vi "getROI.vi"() -> ()   [LabVIEW 2023]
uses:
  <vilib>/vision/NI_Vision_Development_Module.lvlib
panel:
  out "Inverted":T1(plugin-control)
  out "RemoveBorder":T1(plugin-control)
  out "FillHoles":T1(plugin-control)
  out "Threshold":T1(plugin-control)
  in  "Range":cluster{"Lower value":sgl, "Upper value":sgl}={"Lower value"=128.0, "Upper value"=255.0} {"Upper value" format="%.2f"; "Lower value" format="%.2f"}
  out "Ojo Derecho":T1(plugin-control)
  out "error out 3":errorcluster
  out "error out 2":errorcluster
  out "error out":errorcluster
  out "Ojo Izquierdo":T1(plugin-control)
  out "Image 1":T1(plugin-control)
  in  "stop":bool
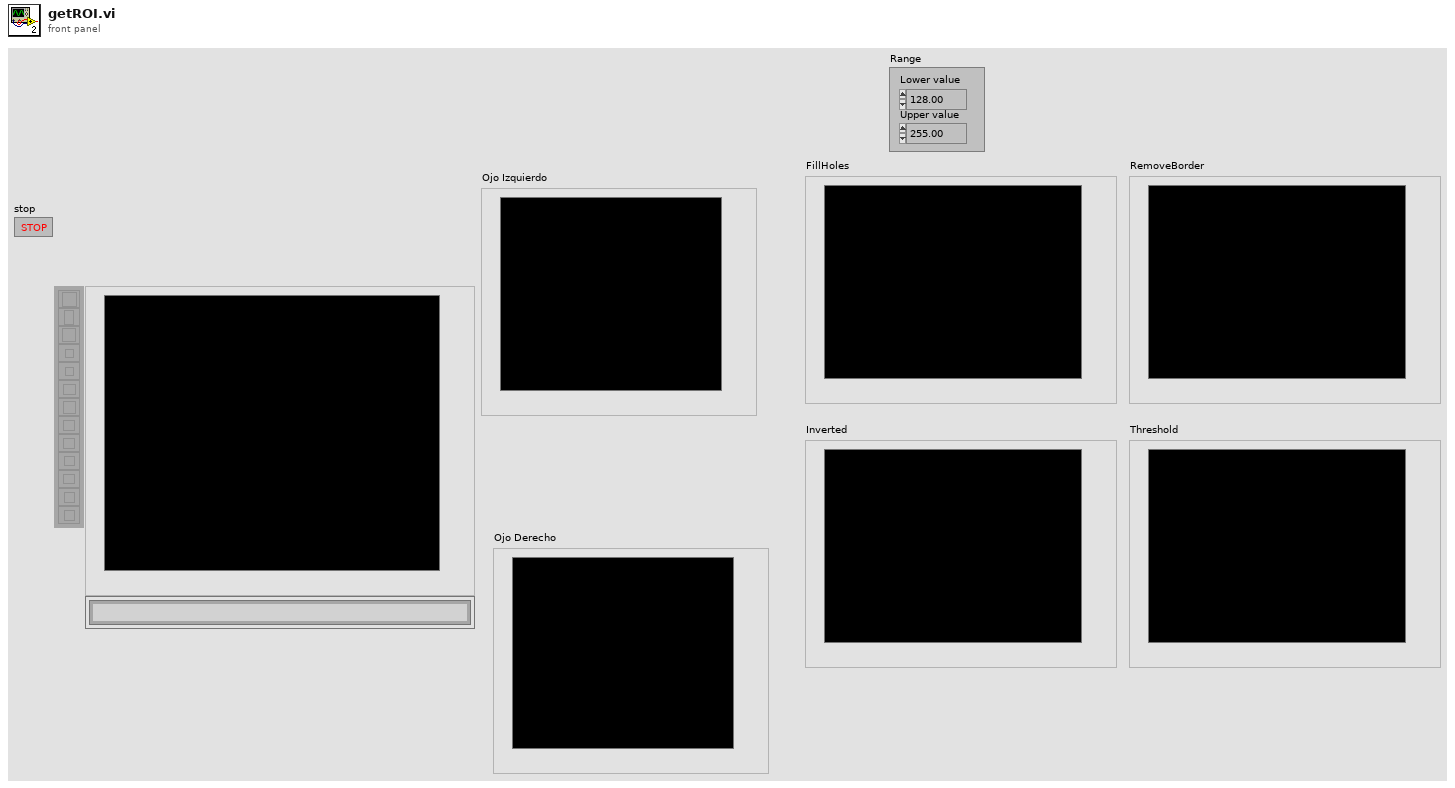
[diagram p1: front panel]
types:
  T1 = typedef "IMAQ Image.ctl" = refnum<image>
  T2 = typedef "Image Type" = u32
  T3 = cluster{"Global Rectangle":i32[], "Contours":cluster{"Contour Type":u32, "ROI Type":u32, "Points":i32[]}[]}
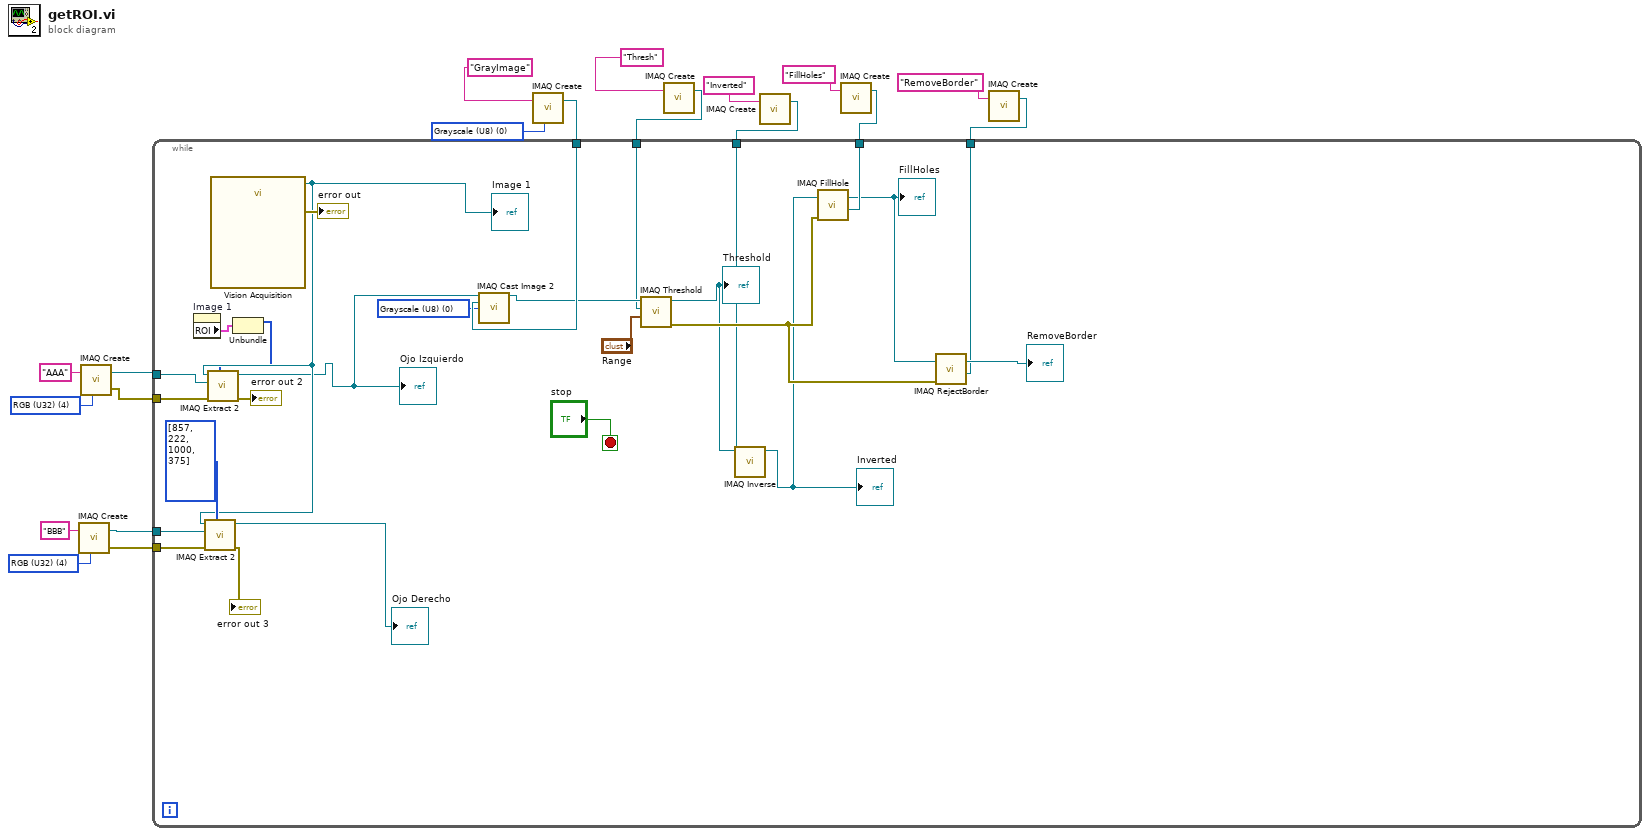
[diagram p0: block diagram]
diagram:
  w9 = T2 0 items=["Grayscale (U8)", "Grayscale (I16)", "Grayscale (SGL)", "Complex (CSG)", "RGB (U32)", "HSL (U32)", "RGB (U64)", "Grayscale (U16)"] ("Image Type")
  w15 = T2 4 items=["Grayscale (U8)", "Grayscale (I16)", "Grayscale (SGL)", "Complex (CSG)", "RGB (U32)", "HSL (U32)", "RGB (U64)", "Grayscale (U16)"] ("Image Type")
  w19 = T2 4 items=["Grayscale (U8)", "Grayscale (I16)", "Grayscale (SGL)", "Complex (CSG)", "RGB (U32)", "HSL (U32)", "RGB (U64)", "Grayscale (U16)"] ("Image Type")
  n1 = call "IMAQ Create"("Image Name"="BBB", "Image Type"=w15) -> ("New Image"=w13:T1, "error out"=w12:errorcluster)  [unwired: 3 in]
  n2 = call "IMAQ Create"("Image Name"="AAA", "Image Type"=w19) -> ("New Image"=w17:T1, "error out"=w16:errorcluster)  [unwired: 3 in]
  n3 = call "IMAQ Create"("Image Name"="GrayImage", "Image Type"=w9) -> ("New Image"=w10:T1)  [unwired: 3 in, 1 out]
  n4 = call "IMAQ Create"("Image Name"="Thresh") -> ("New Image"=w7:T1)  [unwired: 4 in, 1 out]
  n5 = call "IMAQ Create"("Image Name"="Inverted") -> ("New Image"=w1:T1)  [unwired: 4 in, 1 out]
  n6 = call "IMAQ Create"("Image Name"="FillHoles") -> ("New Image"=w5:T1)  [unwired: 4 in, 1 out]
  n7 = call "IMAQ Create"("Image Name"="RemoveBorder") -> ("New Image"=w3:T1)  [unwired: 4 in, 1 out]
  n8 = while {
    tunnel: w17 -> [w42]
    tunnel: w16 -> [w44]
    tunnel: w13 -> [w40]
    tunnel: w12 -> [w39]
    tunnel: w10 -> [w34]
    tunnel: w7 -> [w30]
    tunnel: w5 -> [w27]
    tunnel: w3 -> [w25]
    tunnel: w1 -> [w22]
    stop <- "stop" stop-if-true
    w33 = T2 0 items=["Grayscale (U8)", "Grayscale (I16)", "Grayscale (SGL)", "Complex (CSG)", "RGB (U32)", "HSL (U32)", "RGB (U64)", "Grayscale (U16)"] ("Image Type")
    n9 = property on="Image 1" class="ImageControl"() -> ("ROI"=w29:T3)  [unwired: 2 in, 2 out]
    n10 = call "Vision Acquisition"() -> ("Image Out"=w36:T1, "error out"=→"error out":errorcluster)  [unwired: 25 in, 1 out]
    "Image 1" <- w36
    n11 = call "IMAQ Extract 2"("Optional Rectangle"=i32[] [857, 222, 1000, 375], "error in (no error)"=w39, "Image Dst"=w40, "Image Src"=w36) -> ("error out"=→"error out 3":errorcluster, "Image Dst Out"=→"Ojo Derecho":T1)  [unwired: 6 in]
    n12 = Unbundle(w29) -> ("Global Rectangle"=w28:i32[])  [unwired: 1 out]
    n13 = call "IMAQ Extract 2"("Optional Rectangle"=w28, "error in (no error)"=w44, "Image Dst"=w42, "Image Src"=w36) -> ("error out"=→"error out 2":errorcluster, "Image Dst Out"=w35:T1)  [unwired: 6 in]
    "Ojo Izquierdo" <- w35
    n14 = call "IMAQ Cast Image 2"("Image Src"=w35, "Image Dst"=w34, "Image Type"=w33) -> ("Image Dst Out"=w31:T1)  [unwired: 11 in, 1 out]
    n15 = call "IMAQ Threshold"("Range"="Range", "Image Dst"=w30, "Image Src"=w31) -> ("error out"=w23:errorcluster, "Image Dst Out"=w21:T1)  [unwired: 7 in]
    "Threshold" <- w21
    n16 = call "IMAQ Inverse"("Image Dst"=w22, "Image Src"=w21) -> ("Image Dst Out"=w20:T1)  [unwired: 8 in, 1 out]
    "Inverted" <- w20
    n17 = call "IMAQ FillHole"("error in (no error)"=w23, "Image Dst"=w27, "Image Src"=w20) -> ("Image Dst Out"=w24:T1)  [unwired: 3 in, 1 out]
    "FillHoles" <- w24
    n18 = call "IMAQ RejectBorder"("error in (no error)"=w23, "Image Dst"=w25, "Image Src"=w24) -> ("Image Dst Out"=→"RemoveBorder":T1)  [unwired: 3 in, 1 out]
  }
